vi "Adam_data.vi"() -> ()   [LabVIEW 2018]
panel:
  in  "Vb Moments":cluster{"3":dbl, "2":dbl[], "1":dbl[]}
  in  "Mb Moments":cluster{"1":dbl[], "2":dbl[], "3":dbl}
  in  "Vw Moments":cluster{"3":dbl[], "2":dbl[][], "1":dbl[][]}
  in  "Mw Moments":cluster{"3 ":dbl[], "2":dbl[][], "1":dbl[][]}
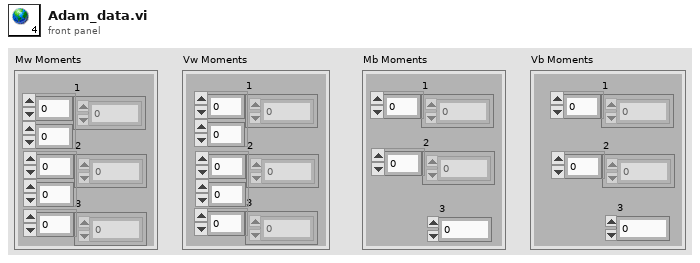
[diagram p1: front panel]
diagram:
